vi "PointMap_Init.vi"(8 "error in (no error)":errorcluster) -> (0 "error out":errorcluster)   [LabVIEW 2017, in "PointValueMap.lvlib"]
doc: "Removes all point value maps and their contents from memory."
uses:
  <vilib>/addons/PointValueMap/PointValueMap.lvlib
  <vilib>/addons/PointValueMap/controls/PointMapOperations.ctl
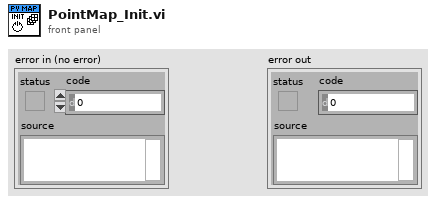
[diagram p1: front panel]
types:
  T1 = typedef "PointValueMap.lvlib/PointMapOperations.ctl" = enum16{"Initialize", "Create Map", "Update Map", "Get Map", "Get All Maps", "Destroy Map", "Destroy All Maps"}
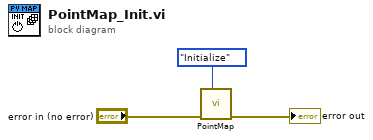
[diagram p0: block diagram]
diagram:
  n1 = call <vilib>:"PointMap.vi"("Operation"=PointMapOperations."Initialize", "error in (no error)"="error in (no error)") -> ("error out"=→"error out":errorcluster)  [unwired: 5 in, 4 out]
